vi "IMU-example.vi"(2 "NXT":T3={"Hardware"="NXT", "Flattened String"=""}, 3 "Input Port":T2=3 caption="Port (Port 4)" items=["Port 1", "Port 2", "Port 3", "Port 4"]) -> (4 "NXT":T3={"Hardware"="NXT", "Flattened String"=""})   [LabVIEW 2010]
doc: "Reads the ultrasonic sensor connected to the specified input port and outputs the distance in centimeters."
uses:
  <vilib>/NXT/Subs/LVHSConnector.ctl
  <vilib>/NXT/Block Support/NXT_InputPort.ctl
  <vilib>/NXT/Mindsensors/Dual/AbsoluteIMU-DM.vi
  <vilib>/NXT/Dual Mode Library/Display/drawNumber.vi
panel:
  in  "Operation":u8(ring) items=["Read Accl", "Read Compass", "Read Magnetic Field", "Read Accl & Compass", "Read Gyro", "Begin Compass Calib", "End Compass Calib", "Sens-2G", "Sens-4G", "Sens-8G", "Sens-16G"]
  out "output cluster":T1
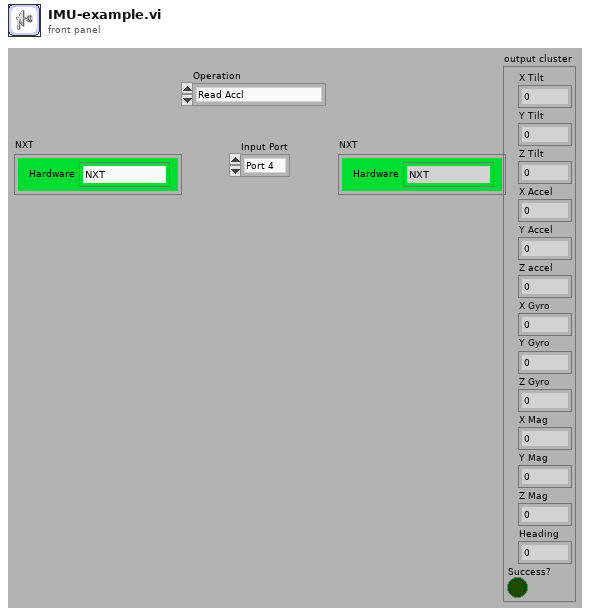
[diagram p1: front panel]
types:
  T1 = cluster{"X Tilt":i32, "Y Tilt":i32, "Z Tilt":i32, "X Accel":i32, "Y Accel":i32, "Z accel":i32, "X Gyro":i32, "Y Gyro":i32, "Z Gyro":i32, "X Mag":i32, "Y Mag":i32, "Z Mag":i32, "Heading":i32, "Success?":bool}
  T2 = typedef "NXT_InputPort.ctl" = u8
  T3 = typedef "LVHSConnector.ctl" = cluster{"Hardware":string, "Flattened String":string}
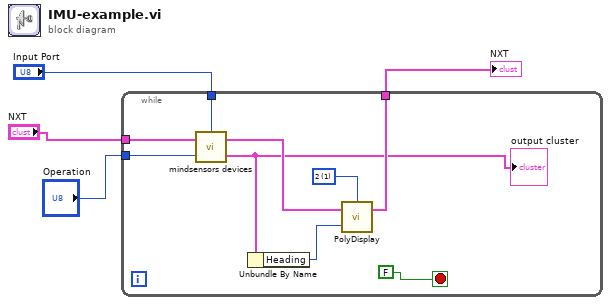
[diagram p0: block diagram]
diagram:
  n1 = while {
    tunnel: "NXT" -> [w13]
    tunnel: "Input Port" -> [w12]
    tunnel: "Operation" -> [w11]
    tunnel: [w10] -> w1
    stop <- FALSE stop-if-true
    w7 = i16 1 items=["1", "2", "3", "4", "5", "6", "7", "8"] ("Line")
    n2 = call-poly <vilib>:"mindsensors devices.vi"("Operation"=w11, "NXT"=w13, "Input Port"=w12) -> ("output cluster"=w5:T1, "NXT dup"=w9:T3)
    "output cluster" <- w5
    n3 = Unbundle By Name(w5) -> ("Heading"=w8:i32)
    n4 = call-poly <vilib>:"PolyDisplay.vi"("number"=w8, "NXT"=w9, "Line"=w7) -> ("NXT"=w10:T3)  [unwired: 1 in]
  }
  "NXT" <- w1
